vi "111-Main.vi"   [LabVIEW 2018]
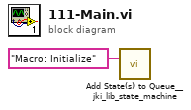
[diagram p0: block diagram]
diagram:
  n1 = call <vilib>:"Add State(s) to Queue__jki_lib_state_machine.vi"("State(s) in (\"\")"="Macro: Initialize") -> ()  [unwired: 14 in, 1 out]
